vi "Read.vi"(8 "error in (no error)":errorcluster, 11 "VeriStand DSF in":refnum<class "VeriStand DSF.lvclass">) -> (0 "error out":errorcluster, 3 "VeriStand DSF out":refnum<class "VeriStand DSF.lvclass">)   [LabVIEW 2020, in "DSF Engine.lvlib" / "VeriStand DSF.lvclass"]
uses:
  VeriStand DSF.lvclass
  Includes/DSF Core.lvlibp/Classes/Framework/Framework.lvclass
  C:/Users/nitest/Desktop/Git/niveristand-data-sharing-framework-custom-device/Includes/DSF Core.lvlibp/Classes/Framework/Framework.lvclass
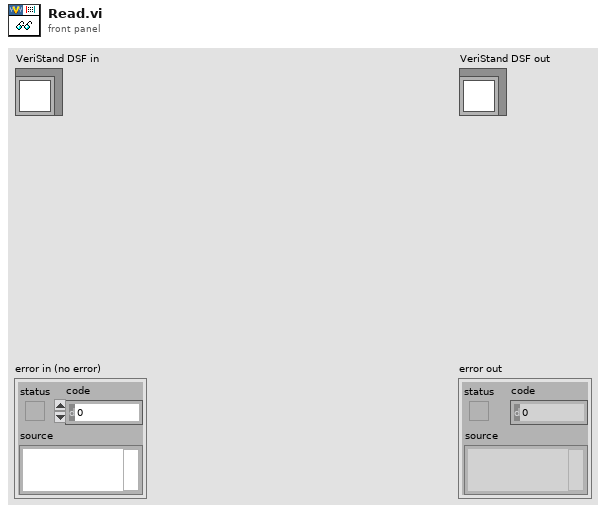
[diagram p1: front panel]
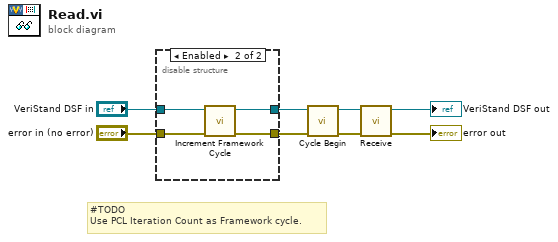
[diagram p0: block diagram]
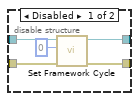
[diagram p2: hidden frame]
diagram:
  # "#TODO\nUse PCL Iteration Count as Framework cycle."
  n1 = disable-structure shown="Enabled" {
    disable-tunnel: "error in (no error)" -> [w13 w16]
    disable-tunnel: "VeriStand DSF in" -> [w12 w17]
    disable-tunnel: [w11 w15] -> w4
    disable-tunnel: [w10 w14] -> w3
    frame Disabled {
      n2 = call "Set Framework Cycle.vi"("error in (no error)"=w13, "iteration"=u64 0, "Framework in"=w12) -> ("error out"=w10:errorcluster, "Framework out"=w11:refnum<class "VeriStand DSF.lvclass">)  [unwired: 7 in]
    }
    frame Enabled {
      n3 = call "Increment Framework Cycle.vi"("error in (no error)"=w16, "Framework in"=w17) -> ("error out"=w14:errorcluster, "Framework out"=w15:refnum<class "VeriStand DSF.lvclass">)  [unwired: 8 in]
    }
  }
  n4 = call "Cycle Begin.vi"("error in (no error)"=w3, "Framework in"=w4) -> ("error out"=w1:errorcluster, "Framework out"=w2:refnum<class "VeriStand DSF.lvclass">)  [unwired: 8 in]
  n5 = call "Receive.vi"("error in"=w1, "framework in"=w2) -> ("error out"=→"error out":errorcluster, "framework out"=→"VeriStand DSF out":refnum<class "VeriStand DSF.lvclass">)  [unwired: 8 in]
